vi "Handle Message.vi"(0 "ICanComunicate In":refnum<class "Process Handler.lvclass">, 7 "Message In":T1, 11 "Error In":errorcluster) -> (4 "ICanComunicate Out":refnum<class "Process Handler.lvclass">, 6 "CMD Out":string, 8 "Message Out":T1, 15 "Error Out":errorcluster)   [LabVIEW 2023, in "Process Handler.lvclass"]
uses:
  Process Handler.lvclass
  Interfaces/ICanCommunicate/Message.ctl
  Interfaces/ICanCommunicate/ICanCommunicate.lvclass
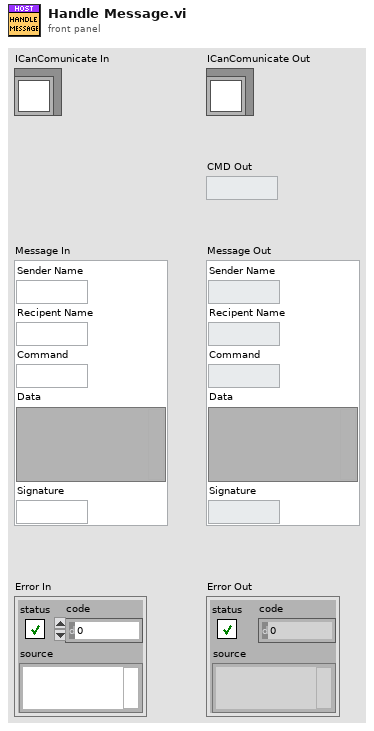
[diagram p1: front panel]
types:
  T1 = typedef "ICanCommunicate.lvclass/Message.ctl" = cluster{"Sender Name":string, "Recipent Name":string, "Command":string, "Data":variant, "Signature":string}
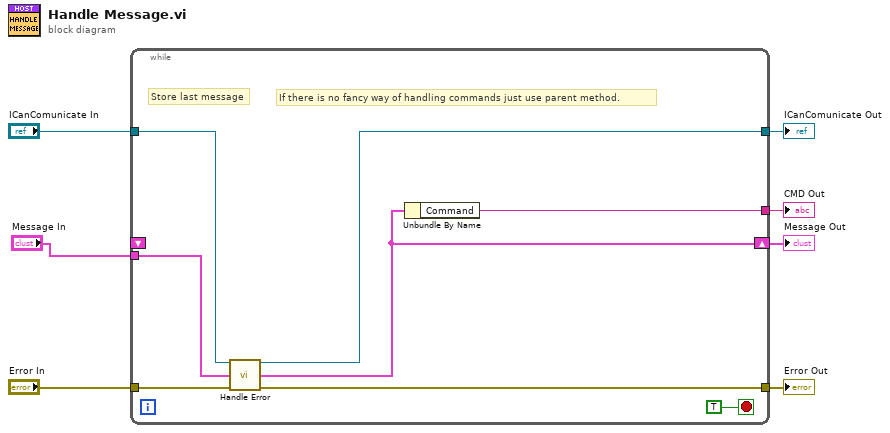
[diagram p0: block diagram]
diagram:
  n1 = while {
    shift-right: [w9] -> w3
    shift-left: _ -> [_]
    tunnel: "Error In" -> [w14]
    tunnel: [w13] -> w6
    tunnel: "ICanComunicate In" -> [w11]
    tunnel: [w10] -> w4
    tunnel: "Message In" -> [w12]
    tunnel: [w8] -> w1
    stop <- TRUE stop-if-true
    # "If there is no fancy way of handling commands just use parent method."
    # "Store last message"
    n2 = call-dynamic "Handle Error.vi"("Process In"=w11, "Message In"=w12, "Error In"=w14) -> ("Process Out"=w10:refnum<class "Process Handler.lvclass">, "Message Out"=w9:T1, "Error Out"=w13:errorcluster)  [unwired: 10 in]
    n3 = Unbundle By Name(w9) -> ("Command"=w8:string)
  }
  "Error Out" <- w6
  "ICanComunicate Out" <- w4
  "Message Out" <- w3
  "CMD Out" <- w1
